vi "Two Button Dialog with Error.vi"(8 "Error In":errorcluster, 9 "F button name (\"Cancel\")":string="Cancel", 10 "T button name (\"OK\")":string="OK", 11 "message":string) -> (0 "Error Out":errorcluster, 2 "T button?":bool)   [LabVIEW 2021, in "GUI.lvlib"]
uses:
  GUI.lvlib
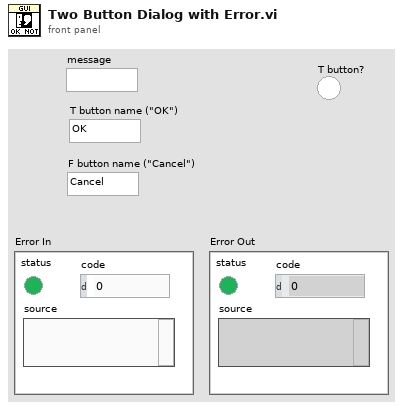
[diagram p1: front panel]
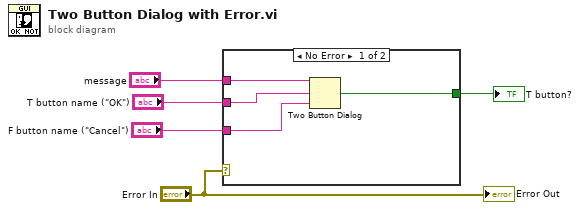
[diagram p0: block diagram]
diagram:
  n1 = case shown="No Error" "Error In" {
    tunnel: "message" -> [w9 _]
    tunnel: "T button name (\"OK\")" -> [w8 _]
    tunnel: "F button name (\"Cancel\")" -> [w7 _]
    tunnel: [w6 _] -> w1
    frame No Error {
      n2 = Two Button Dialog(message=w9, 1:w7, 2:w8) -> (T button?=w6:bool)
    }
    frame Error {
    }
  }
  "T button?" <- w1
  "Error Out" <- "Error In"
